vi "Get Shooter Encoders.vi"() -> (2 "Rate Enc1":dbl, 3 "Rate Enc2":dbl)   [LabVIEW 2015]
panel:
  out "Stopped 2":bool
  out "Stopped":bool
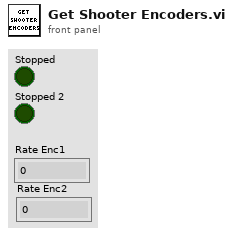
[diagram p1: front panel]
types:
  T1 = typedef "WPI_EncoderDevRef.ctl" = cluster{"DevStatus":errorcluster, "EncoderIndex":T2, "CounterIndex":T3, "DistancePerCount":dbl, "Decoding Type":T4}
  T2 = typedef "FPGA_EncoderIdx.ctl" = enum8{"Enc 0", "Enc 1", "Enc 2", "Enc 3", "Enc 4", "Enc 5", "Enc 6", "Enc 7", "Invalid"}
  T3 = typedef "FPGA_CounterCtrSystemIndex.ctl" = enum8{"Ctr 0", "Ctr 1", "Ctr 2", "Ctr 3", "Ctr 4", "Ctr 5", "Ctr 6", "Ctr 7", "Invalid"}
  T4 = typedef "WPI_EncoderType.ctl" = enum16{"1x", "2x", "4x"}
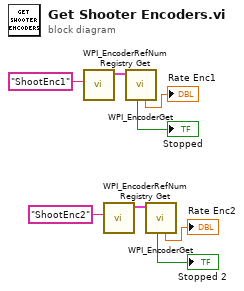
[diagram p0: block diagram]
diagram:
  n1 = call <vilib>:"WPI_EncoderRefNum Registry Get.vi"("refnum name"="ShootEnc1") -> ("EncoderDevRef"=w6:T1)  [unwired: 9 in, 1 out]
  n2 = call <vilib>:"WPI_EncoderRefNum Registry Get.vi"("refnum name"="ShootEnc2") -> ("EncoderDevRef"=w5:T1)  [unwired: 9 in, 1 out]
  n3 = call <vilib>:"WPI_EncoderGet.vi"("EncoderDevRef"=w6) -> ("Rate"=→"Rate Enc1":dbl, "Stopped"=→"Stopped":bool)  [unwired: 5 in, 4 out]
  n4 = call <vilib>:"WPI_EncoderGet.vi"("EncoderDevRef"=w5) -> ("Rate"=→"Rate Enc2":dbl, "Stopped"=→"Stopped 2":bool)  [unwired: 5 in, 4 out]
